vi "get Status As String Array.vi"(11 "Timer in":refnum<class "Timer.lvclass">) -> (3 "Status":string[](array[string]))   [LabVIEW 2015, in "Timer.lvclass"]
uses:
  Timer.lvclass
  Timer.lvclass/Timer.ctl
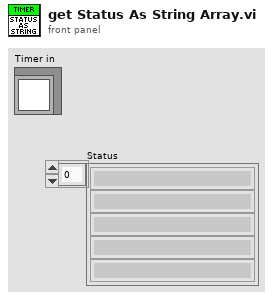
[diagram p1: front panel]
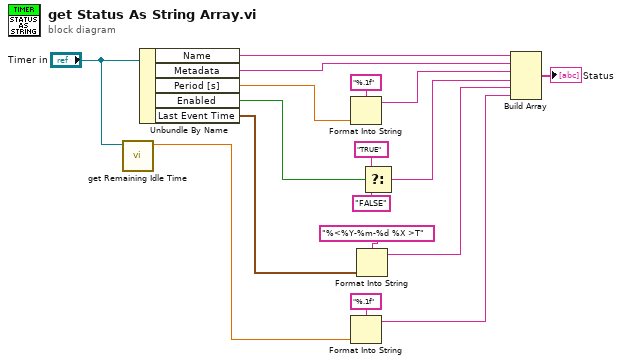
[diagram p0: block diagram]
diagram:
  n1 = call "get Remaining Idle Time.vi"("Timer in"="Timer in") -> ("Remaining Idle Time [s]"=w4:dbl)  [unwired: 10 in]
  n2 = Unbundle By Name("Timer in") -> ("Name"=w16:string, "Metadata"=w1:string, "Period [s]"=w14:dbl, "Enabled"=w10:bool, "Last Event Time"=w7:timestamp)
  n3 = Format Into String(format string="%.1f", w14) -> (resulting string=w13:string)  [unwired: 2 in, 1 out]
  n4 = Format Into String(format string="%.1f", w4) -> (resulting string=w3:string)  [unwired: 2 in, 1 out]
  n5 = Format Into String(format string="%<%Y-%m-%d %X >T", w7) -> (resulting string=w6:string)  [unwired: 2 in, 1 out]
  n6 = Select(t="TRUE", s=w10, f="FALSE") -> (s? t:f=w9:string)
  n7 = Build Array(w16, w1, w13, w9, w6, w3) -> (→"Status":string[])
